vi "Initialize-object.vi"(7 "Heartbeat interval":dbl, 8 "error in (no error)":errorcluster, 9 "Client channel":refnum<queue>, 10 "Server channel":refnum<queue>) -> (0 "error out":errorcluster, 3 "Reference out":T1)   [LabVIEW 2013, in "Client.lvlib" / "Client.lvclass"]
doc: "Initialize the client resources and create a reference to the client object.\n\nRequires initialized communication channels (message queues), one for incoming (client) communication and one for outgoing (server) communication. These are generally intitialized by the 'server' instance which calls the main client vi."
uses:
  Client.lvclass
  Object-reference.ctl
  Messages/Sources/Message.lvclass
  Client.lvclass/Client.ctl
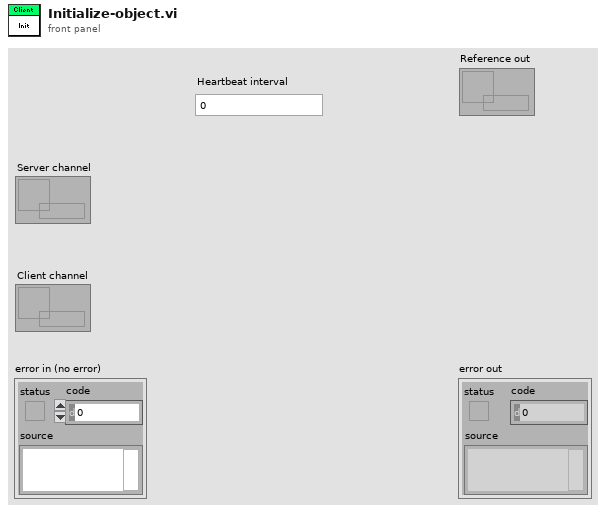
[diagram p1: front panel]
types:
  T1 = typedef "Client.lvlib/Client.lvclass/Object-reference.ctl" = refnum<data-value>
  T2 = typedef "Client.lvlib/Client.lvclass/Supported-modules.ctl" = enum16{"Server", "All", "BeamControl", "PowderDeposition", "StrategyParser", "CameraVision", "MaterialCharacterization", "StatusMonitor", "SLMSimulation", "LaserCharacterization"}
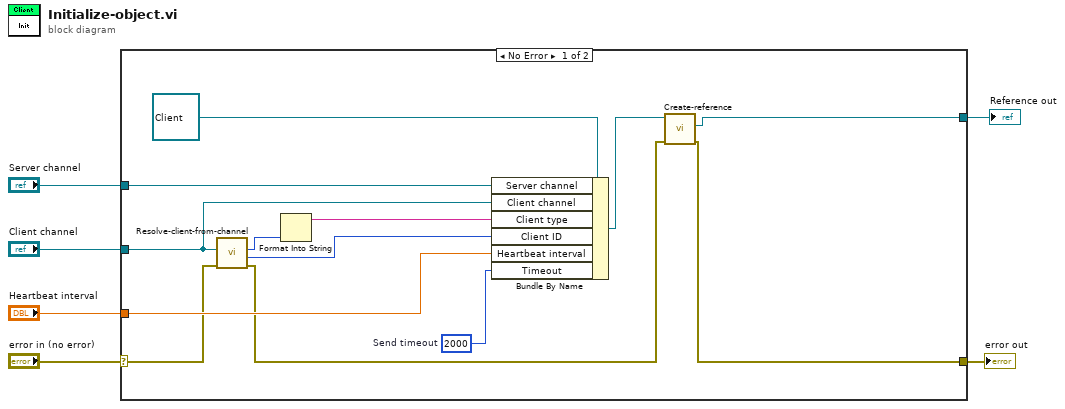
[diagram p0: block diagram]
diagram:
  n1 = case shown="No Error" "error in (no error)" {
    selector: "error in (no error)" -> [w11 w20]
    tunnel: [w19 w20] -> w5
    tunnel: [w18 _] -> w4
    tunnel: "Heartbeat interval" -> [w17 _]
    tunnel: "Client channel" -> [w12 _]
    tunnel: "Server channel" -> [w16 _]
    frame No Error {
      w13 = 2000  # Send timeout
      n2 = call "Resolve-client-from-channel.vi"("error in (no error)"=w11, "Client channel"=w12) -> ("error out"=w10:errorcluster, "Client ID"=w9:i32, "Client type"=w8:T2)  [unwired: 7 in]
      n3 = Format Into String(w8) -> (resulting string=w7:string)  [unwired: 3 in, 1 out]
      n4 = Bundle By Name(cluster=refnum<class "Client.lvclass"> refnum ("Panes.lvclass"), "Server channel"=w16, "Client channel"=w12, "Client type"=w7, "Client ID"=w9, "Heartbeat interval"=w17, "Timeout"=w13) -> (w14:refnum<class "Client.lvclass">)
      n5 = call "Create-reference.vi"("error in (no error)"=w10, "Object in"=w14) -> ("error out"=w19:errorcluster, "Object reference"=w18:T1)  [unwired: 7 in, 1 out]
    }
    frame Error {
    }
  }
  "error out" <- w5
  "Reference out" <- w4
